vi "To Variant.vi"(8 "Error In":errorcluster, 11 "TD Bool A":refnum<class "1D Bool.lvclass">) -> (0 "Error Out":errorcluster, 2 "Variant":variant)   [LabVIEW 2020, in "NI_VIAnCFGDataStructure.lvlib" / "1D Bool.lvclass"]
doc: "Dynamic dispatch interface for conversion of Tree Data classes to variant LV data."
uses:
  <vilib>/addons/analyzer/VIAnCFGDataStructure/Data Types/Bool Array/1D Bool.lvclass
  <vilib>/addons/analyzer/VIAnCFGDataStructure/Data Types/Bool Array/1D Bool.lvclass/1D Bool.ctl
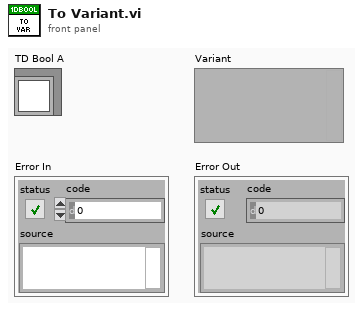
[diagram p1: front panel]
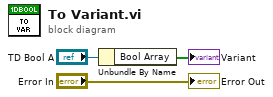
[diagram p0: block diagram]
diagram:
  n1 = Unbundle By Name("TD Bool A") -> ("Bool Array"=→"Variant":bool[])
  "Error Out" <- "Error In"
